vi "SVM Dense Cross-Validate NU_SVR.vi"(6 "Nr fold":i32 caption="Nr fold (LOO)", 7 "Options":T5={"cache_size"=200.0, "eps"=0.001, "shrinking"=TRUE, "probability"=FALSE}, 8 "error in (no error)":errorcluster, 9 "Param NU_SVR":T2={"C"=1.0, "nu"=0.5}, 10 "Kernel":T3, 11 "Dense problem":T1) -> (0 "error out":errorcluster, 3 "Target":dbl[](array[numeric]) caption="Target (Predicted labels)")   [LabVIEW 2015]
doc: "This function conducts cross validation. Data are separated to nr_fold folds. Under given parameters sequentially each fold is validated using the model from training the remaining. Predicted labels (of all prob's instances) in the validation process are stored in the array called target.\n\nThe default number of folds uses Leave-One-Out cross-validation (LOO)."
uses:
  LibSVM Sparse/Controls/Options Training.ctl
  LibSVM Sparse/Controls/Kernel.ctl
  LibSVM Sparse/Wrapper API/Controls/svm_kernel_type.ctl
  LibSVM Sparse/Controls/Parameters NU_SVR.ctl
  Wrapper API/Controls/svmdense_problem.ctl
  LibSVM Sparse/Wrapper API/Controls/svm_parameter.ctl
  LibSVM Sparse/Wrapper API/Controls/svm_type.ctl
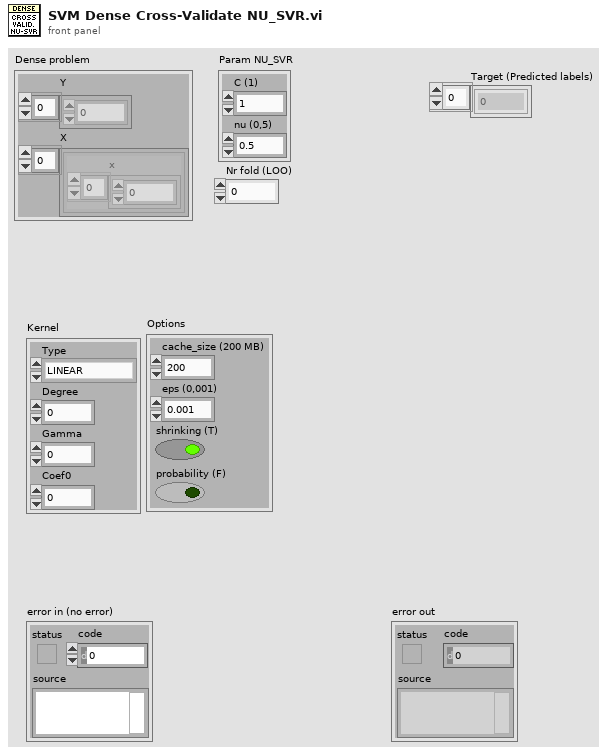
[diagram p1: front panel]
types:
  T1 = typedef "svmdense_problem.ctl" = cluster{"Y":dbl[], "X":cluster{"x":dbl[]}[]}
  T2 = typedef "Parameters NU_SVR.ctl" = cluster{"C":dbl, "nu":dbl}
  T3 = typedef "Kernel.ctl" = cluster{"Type":T4, "Degree":i32, "Gamma":dbl, "Coef0":dbl}
  T4 = typedef "svm_kernel_type.ctl" = enum32{"LINEAR", "POLY", "RBF", "SIGMOID", "PRECOMPUTED"}
  T5 = typedef "Options Training.ctl" = cluster{"cache_size":dbl, "eps":dbl, "shrinking":bool, "probability":bool}
  T6 = typedef "svm_type.ctl" = enum32{"C_SVC", "NU_SVC", "ONE_CLASS", "EPSILON_SVR", "NU_SVR"}
  T7 = typedef "svm_parameter.ctl" = cluster{"svm_type":T6, "kernel_type":T4, "degree":i32, "gamma":dbl, "coef0":dbl, "cache_size":dbl, "eps":dbl, "C":dbl, "weight_label":i32[], "weight":dbl[], "nu":dbl, "p":dbl, "shrinking":bool, "probability":bool}
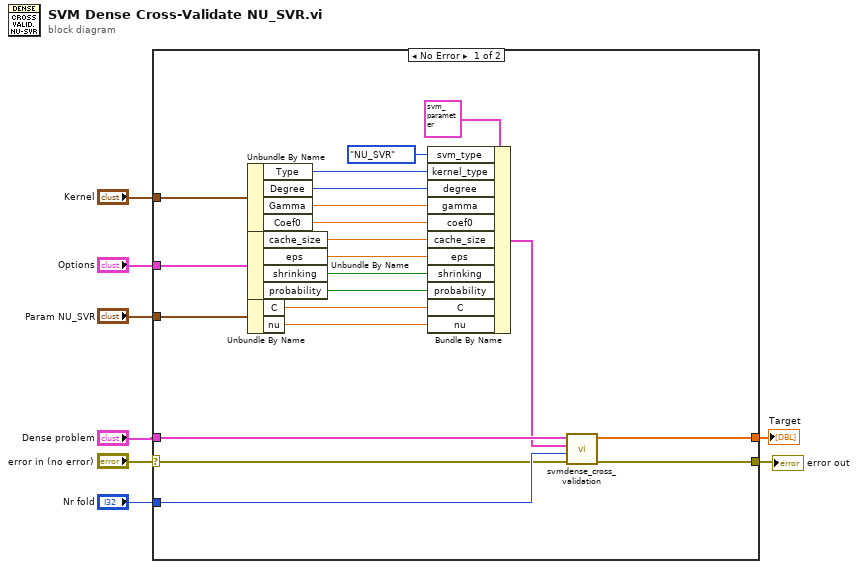
[diagram p0: block diagram]
diagram:
  n1 = case shown="No Error" "error in (no error)" {
    selector: "error in (no error)" -> [w11 w30]
    tunnel: [w10 w30] -> w8
    tunnel: "Dense problem" -> [w14 _]
    tunnel: "Kernel" -> [w28 _]
    tunnel: [w9 _] -> w3
    tunnel: "Options" -> [w19 _]
    tunnel: "Param NU_SVR" -> [w20 _]
    tunnel: "Nr fold" -> [w12 _]
    frame No Error {
      n2 = Unbundle By Name(w28) -> ("Type"=w27:T4, "Degree"=w26:i32, "Gamma"=w25:dbl, "Coef0"=w24:dbl)
      n3 = Unbundle By Name(w19) -> ("cache_size"=w22:dbl, "eps"=w21:dbl, "shrinking"=w18:bool, "probability"=w17:bool)
      n4 = Unbundle By Name(w20) -> ("C"=w16:dbl, "nu"=w15:dbl)
      n5 = Bundle By Name(cluster=T7 {"svm_type"=enum."C_SVC", "kernel_type"=enum."LINEAR", "degree"=0, "gamma"=0.0, "coef0"=0.0, "cache_size"=0.0, "eps"=0.0, "C"=0.0, "weight_label"=[], "weight"=[], "nu"=0.0, "p"=0.0, "shrinking"=FALSE, "probability"=FALSE} ("svm_parameter"), "svm_type"=svm_type."NU_SVR", "kernel_type"=w27, "degree"=w26, "gamma"=w25, "coef0"=w24, "cache_size"=w22, "eps"=w21, "shrinking"=w18, "probability"=w17, "C"=w16, "nu"=w15) -> (w13:T7)
      n6 = call "svmdense_cross_validation.vi"("error in (no error)"=w11, "Nr fold"=w12, "Parameters"=w13, "Problem"=w14) -> ("error out"=w10:errorcluster, "Target"=w9:dbl[])  [unwired: 6 in]
    }
    frame Error {
    }
  }
  "error out" <- w8
  "Target" <- w3
